vi "BooleanRise.vi"(8 "error in (no error)":errorcluster, 10 "Boolean in":bool, 11 "Utilities in":refnum<class "Utilities.lvclass">) -> (0 "error out":errorcluster, 2 "Boolean":bool, 3 "Utilities out":refnum<class "Utilities.lvclass">)   [LabVIEW 2020, in "Utilities.lvclass"]
uses:
  Utilities.lvclass
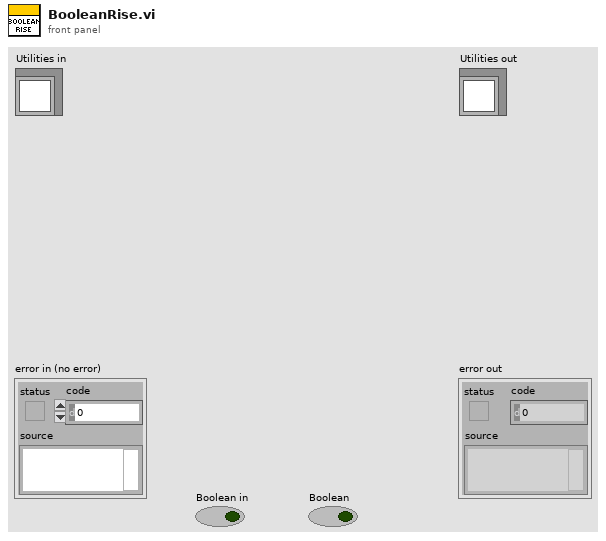
[diagram p1: front panel]
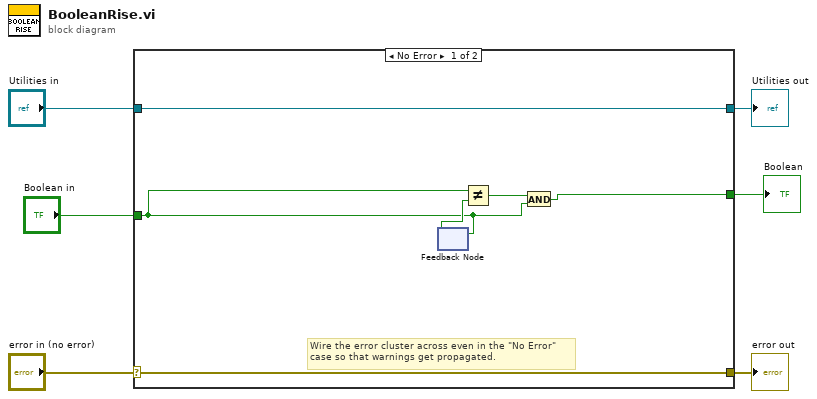
[diagram p0: block diagram]
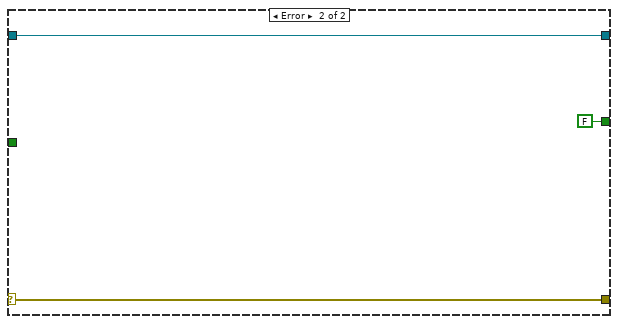
[diagram p2: hidden frame]
diagram:
  n1 = case shown="No Error" "error in (no error)" {
    selector: "error in (no error)" -> [w11 w15]
    tunnel: [w11 w15] -> w5
    tunnel: [w12 w14] -> w3
    tunnel: "Utilities in" -> [w12 w14]
    tunnel: "Boolean in" -> [w8 _]
    tunnel: [w7 FALSE] -> w1
    frame No Error {
      # "Wire the error cluster across even in the \"No Error\"\ncase so that warnings get propagated."
      n2 = feedback #1() -> (w9:bool)  [unwired: 1 in]
      n3 = feedback-in #1(w8) -> ()
      n4 = Not Equal?(x=w8, y=w9) -> (x != y?=w10:bool)
      n5 = And(x=w10, y=w8) -> (x .and. y?=w7:bool)
    }
    frame Error {
    }
  }
  "error out" <- w5
  "Utilities out" <- w3
  "Boolean" <- w1
